vi "SRV_ddddd String to Sensor View Indicator Name.vi"(7 "ddddd":string, 11 "error in (no error)":errorcluster) -> (8 "Sensor View Indicator Names":T1, 15 "error out":errorcluster)   [LabVIEW 2014]
uses:
  SRV_Sensors Names.ctl
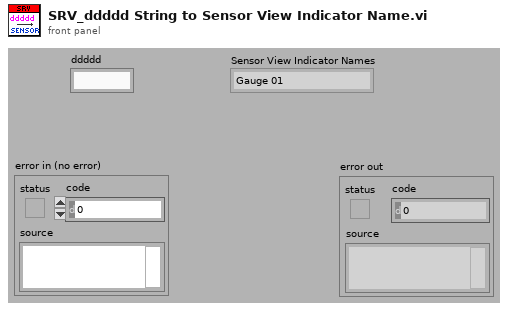
[diagram p1: front panel]
types:
  T1 = typedef "SRV_Sensors Names.ctl" = enum16{"Gauge 01", "Gauge 02", "Gauge 03", "Gauge 04", "Meter 01", "Meter 02", "Meter 03", "Meter 04", "Numeric 01", "Numeric 02", "Numeric 03", "Numeric 04", "Numeric 05", "Numeric 06", "Numeric 07", "Numeric 08", "Boolean 01", "Boolean 02", "Boolean 03", "Boolean 04", "Boolean 05", "Boolean 06", "Boolean 07", "Boolean 08", "Boolean 09", "Boolean 10", "Boolean 11", "Boolean 12", "Boolean 13", "Boolean 14", "Boolean 15", "Boolean 16", "Boolean 17", "Boolean 18", "Boolean 19", "Boolean 20", "Boolean 21", "Boolean 22", "Boolean 23", "Boolean 24", "Boolean 25", "Boolean 26", "Boolean 27", "Boolean 28", "Boolean 29", "Boolean 30", "Boolean 31", "Boolean 32"}
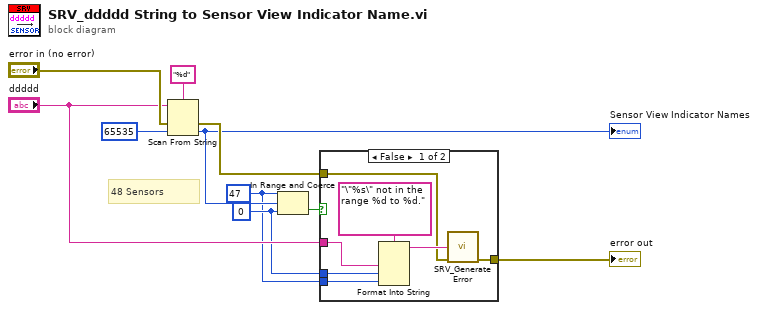
[diagram p0: block diagram]
diagram:
  w1 = u16 47 ("upper limit")
  w2 = u16 0 ("lower limit")
  # "48 Sensors"
  n1 = Scan From String(format string="%d", input string="ddddd", error in="error in (no error)", default 1=u16 65535) -> (error out=w5:errorcluster, output 1=w3:u16)  [unwired: 1 in, 2 out]
  "Sensor View Indicator Names" <- w3
  n2 = In Range and Coerce(upper limit=w1, x=w3, lower limit=w2) -> (In Range?=w4:bool)  [unwired: 1 out]
  n3 = case shown="False" w4 {
    tunnel: w5 -> [w13 w18]
    tunnel: [w17 w18] -> w8
    tunnel: "ddddd" -> [w16 _]
    tunnel: w2 -> [w12 _]
    tunnel: w1 -> [w11 _]
    frame False {
      n4 = Format Into String(format string="\"%s\" not in the range %d to %d.", w16, w12, w11) -> (resulting string=w15:string)  [unwired: 2 in, 1 out]
      n5 = call "SRV_Generate Error.vi"("Message"=w15, "error in (no error)"=w13) -> ("error out"=w17:errorcluster)  [unwired: 13 in]
    }
    frame True {
    }
  }
  "error out" <- w8
